vi "Add System.vi"(8 "error in (no error)":errorcluster, 11 "Manager in":refnum<class "Manager.lvclass">) -> (0 "error out":errorcluster, 3 "Manager out":refnum<class "Manager.lvclass">)   [LabVIEW 2012, in "Manager.lvlib" / "Manager.lvclass"]
uses:
  Manager.lvclass
  <vilib>/ActorFramework/Actor/Actor.lvclass
  Bioreactor Actor/Bioreactor/Bioreactor.lvclass
  <vilib>/Instr/_visa.llb/VISA Configure Serial Port (Instr).vi
  Manager Messages/Update SubPanel Msg/Update SubPanel Msg.lvclass
  Time Protocol Actor/Time Protocol/Time Protocol.lvclass
  Python Protocol Actor/Python Protocol/Python Protocol.lvclass
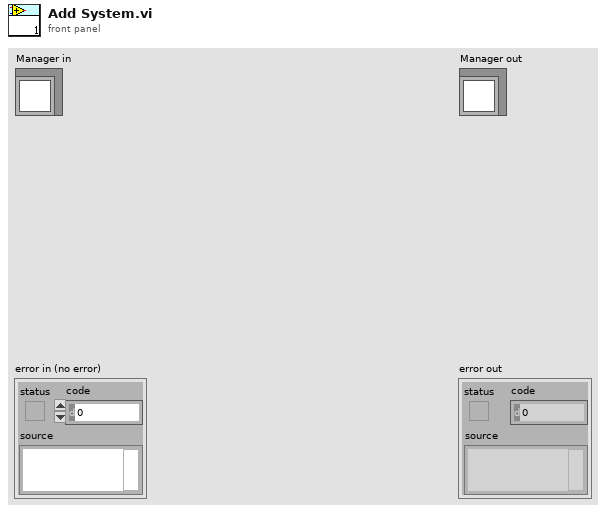
[diagram p1: front panel]
types:
  T1 = enum16{"open", "open or create", "create or replace", "create", "open (read-only)"}
  T2 = cluster{"Bioreactor Queue":refnum<class "Message Enqueuer.lvclass">, "Time Protocol Queue":refnum<class "Message Enqueuer.lvclass">, "Python Protocol Queue":refnum<class "Message Enqueuer.lvclass">, "Name":string}[]
  T3 = cluster{"Caller-To-Actor Enqueuer":refnum<class "Message Enqueuer.lvclass">, "Caller-To-Actor Enqueuer":refnum<class "Message Enqueuer.lvclass">, "Caller-To-Actor Enqueuer":refnum<class "Message Enqueuer.lvclass">, "Name":string}
  T4 = cluster{"Caller-To-Actor Enqueuer":refnum<class "Message Enqueuer.lvclass">, "Caller-To-Actor Enqueuer":refnum<class "Message Enqueuer.lvclass">, "Caller-To-Actor Enqueuer":refnum<class "Message Enqueuer.lvclass">, "Name":string}[]
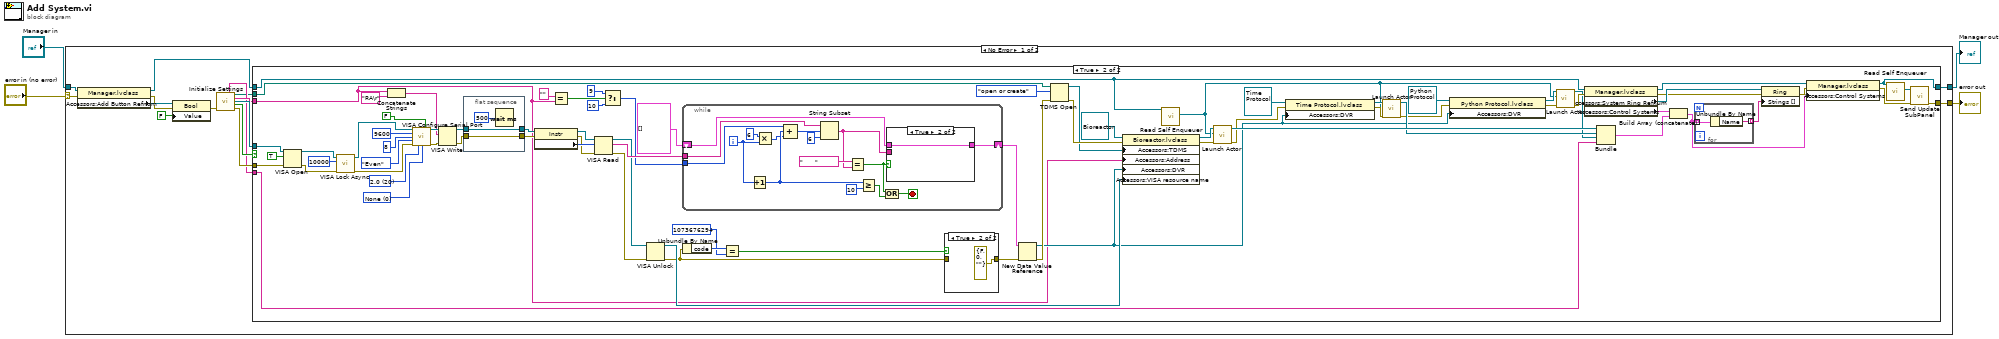
[diagram p0: block diagram]
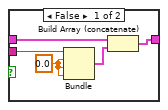
[diagram p3: hidden frame]
diagram:
  n1 = case shown="No Error" "error in (no error)" {
    selector: "error in (no error)" -> [w11 w130]
    tunnel: [w19 w130] -> w3
    tunnel: [w15 w129] -> w1
    tunnel: "Manager in" -> [w9 w129]
    frame No Error {
      n2 = property class="Manager.lvclass"(reference=w9, error in=w11) -> (reference out=w8:refnum<class "Manager.lvclass">, error out=w12:errorcluster, "Accessors:Add Button Refnum"=w14:refnum<vi>)
      n3 = property class="Bool"(reference=w14, error in=w12, "Value"=FALSE ("duplicate session (F)")) -> (error out=w10:errorcluster)  [unwired: 1 out]
      n4 = call "Initialize Settings.vi"("error in (no error)"=w10) -> ("Name"=w6:string, "Data File Path 2"=w5:path, "Address"=w7:string, "Comm Port"=w17:refnum<visa-resource-name>, "bool"=w16:bool, "error out"=w18:errorcluster)  [unwired: 9 in]
      n5 = case shown="True" w16 {
        tunnel: [w21 w50] -> w19
        tunnel: w18 -> [w21 w82]
        tunnel: w17 -> [_ w81]
        tunnel: w7 -> [_ w28]
        tunnel: w8 -> [w20 w88]
        tunnel: w6 -> [_ w43]
        tunnel: [w20 w53] -> w15
        tunnel: w5 -> [_ w54]
        frame False {
        }
        frame True {
          w94 = u16 0 items=["None", "XON/XOFF", "RTS/CTS", "XON/XOFF & RTS/CTS", "DTR/DSR", "XON/XOFF & DTR/DSR"] ("flow control (0:none)")
          w95 = u16 20 items=["1.0"=10, "1.5"=15, "2.0"=20] ("stop bits (10: 1 bit)")
          n6 = VISA Open(duplicate session (F)=TRUE, error in (no error)=w82, VISA resource name=w81) -> (VISA resource name=w79:refnum<visa-resource-name>, error out=w77:errorcluster)  [unwired: 2 in]
          n7 = call <vilib>:"VISA Lock Async.vi"("error in (no error)"=w77, "timeout (0)"=u32 10000, "VISA resource name"=w79) -> ("error out"=w76:errorcluster, "VISA resource name out"=w78:refnum<visa-resource-name>)  [unwired: 6 in, 1 out]
          n8 = Concatenate Strings(w28, "RA\r") -> (w66:string)
          n9 = call-poly "VISA Configure Serial Port"("VISA resource name"=w78, "Enable Termination\nChar (T)"=FALSE ("Enable Termination Char (T)"), "baud rate (9600)"=9600, "data bits (8)"=8, "parity (0:none)"=enum16{"None", "Odd", "Even", "Mark", "Space"}."Even", "error in (no error)"=w76, "stop bits (10: 1 bit)"=w95, "flow control (0:none)"=w94) -> ("VISA resource name out"=w83:refnum<visa-resource-name>, "error out"=w84:errorcluster)  [unwired: 1 in, 5 out]
          n10 = VISA Write(VISA resource name=w83, write buffer=w66, error in (no error)=w84) -> (VISA resource name out=w71:refnum<visa-resource-name>, error out=w69:errorcluster)  [unwired: 1 out]
          n11 = flat-sequence {
            tunnel: [w128] -> w70
            tunnel: w71 -> [w128]
            tunnel: [w127] -> w68
            tunnel: w69 -> [w127]
            frame #0 {
              n12 = Wait (ms)(milliseconds to wait=500 ("y")) -> ()  [unwired: 1 out]
            }
          }
          n13 = property class="Instr"(reference=w70, error in=w68) -> (reference out=w72:refnum<visa-resource-name>, error out=w73:errorcluster, "Serial Settings:Number of Bytes at Serial Port"=w74:u32)
          n14 = Equal?(x="", y=w28) -> (x = y?=w29:bool)
          n15 = VISA Read(VISA resource name=w72, byte count=w74, error in (no error)=w73) -> (VISA resource name out=w61:refnum<visa-resource-name>, read buffer=w62:string, error out=w60:errorcluster)  [unwired: 1 out]
          n16 = Select(t=9, s=w29, f=10) -> (s? t:f=w24:i32)
          n17 = VISA Unlock(8:w60, 11:w61) -> (0:w59:errorcluster, 3:w89:refnum<visa-resource-name>)
          n18 = while {
            tunnel: w62 -> [w117]
            tunnel: w24 -> [w116]
            shift-right: [w102] -> w22
            shift-left: cluster{"read buffer":string, dbl, dbl, dbl}[] [] -> [w103]
            i -> [w107]
            stop <- w111 stop-if-true
            n19 = Increment(x=w107) -> (x+1=w114:i32)
            n20 = Multiply(x=6, y=w107) -> (x*y=w106:i32)
            n21 = Compound Arithmetic op=ADD(w116, w114, w106) -> (w115:i32)
            n22 = String Subset(string=w117, offset (0)=w115, length (rest)=6) -> (substring=w109:string)
            n23 = Equal?(x="      " ("y"), y=w109) -> (x = y?=w104:bool)
            n24 = Greater Or Equal?(x=w114, y=10) -> (x >= y?=w112:bool)
            n25 = Or(x=w104, y=w112) -> (x .or. y?=w111:bool)
            n26 = case shown="True" w104 {
              tunnel: w109 -> [w122 _]
              tunnel: w103 -> [w120 w123]
              tunnel: [w118 w123] -> w102
              frame False {
                w121 = 0.0
                n27 = Bundle("read buffer"=w122, w121, w121, w121) -> (w119:cluster{"read buffer":string, dbl, dbl, dbl})  [unwired: 1 in]
                n28 = Build Array (concatenate)(w120, w119) -> (w118:cluster{"read buffer":string, dbl, dbl, dbl}[])
              }
              frame True {
              }
            }
          }
          n29 = Unbundle By Name(w59) -> ("code"=w65:i32)
          n30 = Equal?(x=w65, y=1073676294) -> (x = y?=w63:bool)
          n31 = case shown="True" w63 {
            tunnel: w59 -> [w124 _]
            tunnel: [w124 errorcluster {"status"=FALSE, "code"=0, "source"=""} ("error constant")] -> w90
            frame False {
            }
            frame True {
            }
          }
          n32 = New Data Value Reference(data value=w22, error in=w90) -> (data value reference=w33:refnum<data-value>, error out=w57:errorcluster)
          n33 = TDMS Open(8:w57, 10:T1."open or create" ("operation"), 11:w54) -> (0:w56:errorcluster, 3:w55:refnum<k34>)  [unwired: 3 in]
          n34 = property class="Bioreactor.lvclass"(reference=refnum<class "Bioreactor.lvclass"> refnum ("Bioreactor Actor.lvlib:Bioreactor.lvclass"), error in=w56, "Accessors:TDMS"=w55, "Accessors:Address"=w28, "Accessors:DVR"=w33, "Accessors:VISA resource name"=w89) -> (reference out=w91:refnum<class "Bioreactor.lvclass">, error out=w93:errorcluster)
          n35 = call <vilib>:"Read Self Enqueuer.vi"("Actor"=w88) -> ("Self Enqueuer"=w32:refnum<class "Message Enqueuer.lvclass">)  [unwired: 10 in]
          n36 = call <vilib>:"Launch Actor.vi"("error in (no error)"=w93, "Actor-to-Caller Enqueuer"=w32, "Actor"=w91) -> ("error out"=w40:errorcluster, "Caller-To-Actor Enqueuer"=w87:refnum<class "Message Enqueuer.lvclass">)  [unwired: 7 in]
          n37 = property class="Time Protocol.lvclass"(reference=refnum<class "Time Protocol.lvclass"> refnum ("Time Protocol Actor.lvlib:Time Protocol.lvclass"), error in=w40, "Accessors:DVR"=w33) -> (reference out=w39:refnum<class "Time Protocol.lvclass">, error out=w41:errorcluster)
          n38 = call <vilib>:"Launch Actor.vi"("error in (no error)"=w41, "Actor-to-Caller Enqueuer"=w32, "Actor"=w39) -> ("error out"=w34:errorcluster, "Caller-To-Actor Enqueuer"=w38:refnum<class "Message Enqueuer.lvclass">)  [unwired: 7 in]
          n39 = property class="Python Protocol.lvclass"(reference=refnum<class "Python Protocol.lvclass"> refnum ("Python Protocol Actor.lvlib:Python Protocol.lvclass"), error in=w34, "Accessors:DVR"=w33) -> (reference out=w37:refnum<class "Python Protocol.lvclass">, error out=w36:errorcluster)
          n40 = call <vilib>:"Launch Actor.vi"("error in (no error)"=w36, "Actor-to-Caller Enqueuer"=w32, "Actor"=w37) -> ("error out"=w31:errorcluster, "Caller-To-Actor Enqueuer"=w30:refnum<class "Message Enqueuer.lvclass">)  [unwired: 7 in]
          n41 = property class="Manager.lvclass"(reference=w88, error in=w31) -> (reference out=w85:refnum<class "Manager.lvclass">, error out=w47:errorcluster, "Accessors:System Ring Refnum"=w48:refnum<vi>, "Accessors:Control Systems"=w49:T2)
          n42 = Bundle("Caller-To-Actor Enqueuer"=w87, "Caller-To-Actor Enqueuer"=w38, "Caller-To-Actor Enqueuer"=w30, "Name"=w43) -> (w86:T3)  [unwired: 1 in]
          n43 = Build Array (concatenate)(w49, w86) -> (w45:T4)
          n44 = for {
            tunnel: w45 -> [w101] mode=indexing
            tunnel: [w100] -> w44 mode=indexing
            n45 = Unbundle By Name(w101) -> ("Name"=w100:string)
          }
          n46 = property class="Ring"(reference=w48, error in=w47, "Strings []"=w44) -> (error out=w46:errorcluster)  [unwired: 1 out]
          n47 = property class="Manager.lvclass"(reference=w85, error in=w46, "Accessors:Control Systems"=w45) -> (reference out=w53:refnum<class "Manager.lvclass">, error out=w51:errorcluster)
          n48 = call <vilib>:"Read Self Enqueuer.vi"("Actor"=w53) -> ("Self Enqueuer"=w52:refnum<class "Message Enqueuer.lvclass">)  [unwired: 10 in]
          n49 = call "Send Update SubPanel.vi"("error in (no error)"=w51, "Message Enqueuer"=w52) -> ("error out"=w50:errorcluster)  [unwired: 8 in, 1 out]
        }
      }
    }
    frame Error {
    }
  }
  "error out" <- w3
  "Manager out" <- w1
